vi "9213_UI.vi"(8 "error in (no error)":errorcluster, 11 "Node Ptr":T5 format="%.0x") -> (0 "error out":errorcluster)   [LabVIEW 2019, in "Modules.lvlib" / "9213.lvclass"]
uses:
  9213.lvclass
  <vilib>/NI VeriStand/Custom Device API/Custom Device Item Ref.ctl
  RSI Module/SubPanel Command.ctl
  Channels Listbox.ctl
  Thermocouple Type.ctl
  Measurement Units.ctl
  Conversion Time.ctl
  C:/Users/nitest/Desktop/Git 2019/niveristand-scan-engine-module-libraries/Source/RSI Module/RSI Module.lvclass
  9213.lvclass/9213.ctl
  RSI Module/RSI Module.lvclass
  <vilib>/NI VeriStand/Custom Device API/Custom Device API.lvlib
panel:
  in  "OTDComp":bool
  in  "Conversion Time":T1=1 items=["High Speed", "High Resolution"]
  in  "Units":T2 caption="Measurement Units" items=["Raw Volts", "Degrees Kelvin", "Degrees Celsius", "Degrees Fahrenheit", "Degrees Rankine"]
  in  "Type":T3 caption="Thermocouple Type" items=["J", "K", "T", "E", "R", "S", "N", "B"]
  in  "Channels":T4=[0]
  in  "SubPanel Event":refnum<user-event>
  in  "Header":cluster{"Section Name":string}={"Section Name"="NI 9205 Settings"}
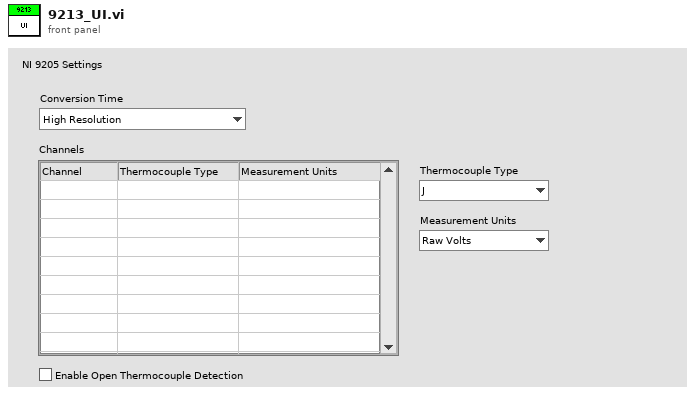
[diagram p1: front panel]
types:
  T1 = typedef "Modules.lvlib/9213.lvclass/Conversion Time.ctl" = u16
  T2 = typedef "Modules.lvlib/9213.lvclass/Measurement Units.ctl" = u8
  T3 = typedef "Modules.lvlib/9213.lvclass/Thermocouple Type.ctl" = u8
  T4 = typedef "Modules.lvlib/9213.lvclass/Channels Listbox.ctl" = i32[]
  T5 = typedef "Custom Device API.lvlib/Custom Device Item Ref.ctl" = u64
  T6 = typedef "Modules.lvlib/RSI Module.lvclass/Module Models.ctl" = enum16{"Empty", "NI 9201", "NI 9203", "NI 9205", "NI 9206", "NI 9207", "NI 9208", "NI 9209", "NI 9210", "NI 9211", "NI 9212", "NI 9213", "NI 9214", "NI 9215", "NI 9216", "NI 9217", "NI 9219", "NI 9220", "NI 9221", "NI 9222", "NI 9223", "NI 9224", "NI 9225", "NI 9226", "NI 9227", "NI 9228", "NI 9229", "NI 9233", "NI 9234", "NI 9235", "NI 9236", "NI 9237", "NI 9239", "NI 9242", "NI 9244", "NI 9253", "NI 9263", "NI 9264", "NI 9265", "NI 9266", "NI 9269", "NI 9344", "NI 9350", "NI 9375", "NI 9401", "NI 9402", "NI 9403", "NI 9411", "NI 9421", "NI 9422", "NI 9423", "NI 9425", "NI 9426", "NI 9435", "NI 9436", "NI 9437", "NI 9472", "NI 9474", "NI 9475", "NI 9476", "NI 9477", "NI 9478", "NI 9481", "NI 9482", "NI 9485"}
  T7 = typedef "Modules.lvlib/RSI Module.lvclass/SubPanel Command.ctl" = enum16{"Stop"}
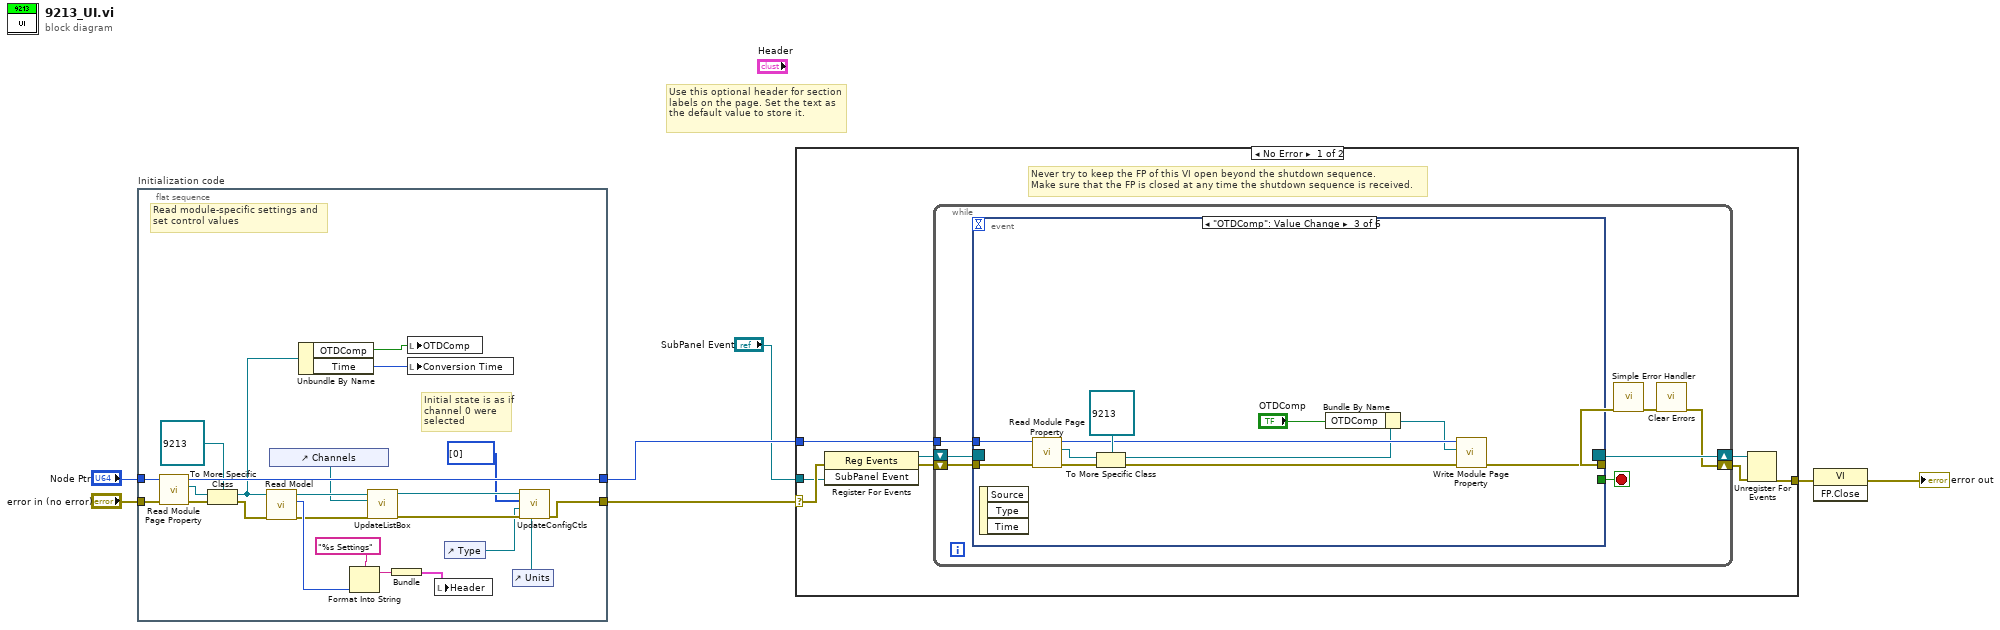
[diagram p0: block diagram]
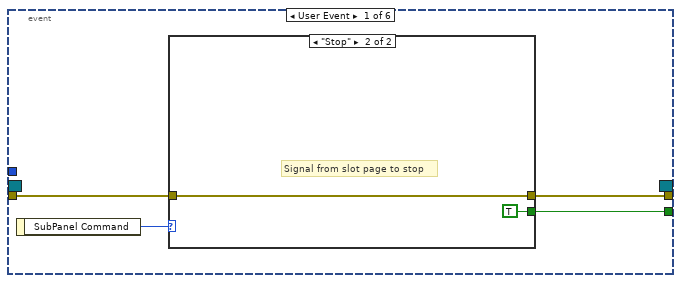
[diagram p2: hidden frame]
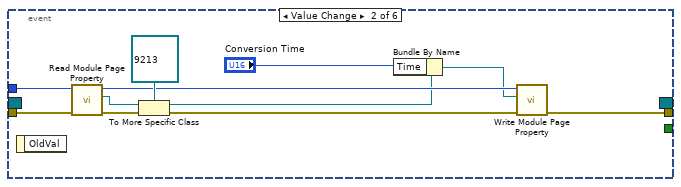
[diagram p4: hidden frame]
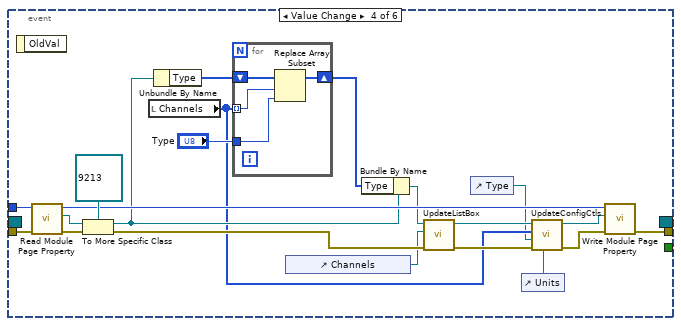
[diagram p5: hidden frame]
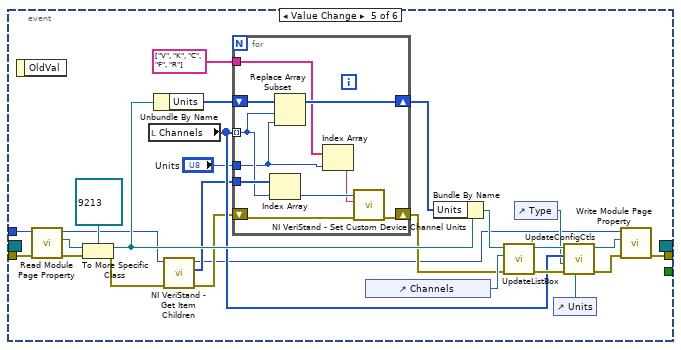
[diagram p6: hidden frame]
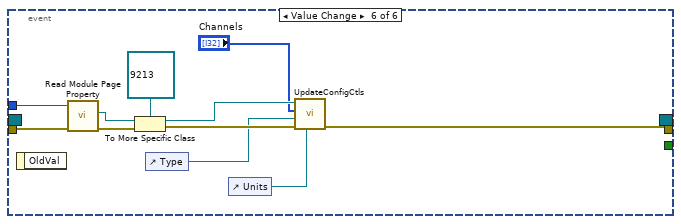
[diagram p7: hidden frame]
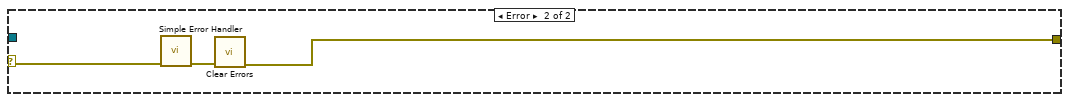
[diagram p8: hidden frame]
diagram:
  # "Use this optional header for section labels on the page. Set the text as the default value to store it."
  n1 = flat-sequence "Initialization code" {
    tunnel: "error in (no error)" -> [w29]
    tunnel: "Node Ptr" -> [w30]
    tunnel: [w12] -> w1
    tunnel: [w28] -> w4
    frame #0 {
      # "Initial state is as if channel 0 were selected"
      # "Read module-specific settings and\nset control values"
      n2 = call "Read Module Page Property.vi"("error in (no error)"=w29, "Node Ptr In"=w30) -> ("error out"=w27:errorcluster, "RSI Module"=w25:refnum<class "RSI Module.lvclass">, "Node Ptr Out"=w28:T5)  [unwired: 7 in]
      n3 = To More Specific Class(target class=refnum<class "9213.lvclass"> refnum ("9205 in"), reference=w25, error in=w27) -> (specific class reference=w15:refnum<class "9213.lvclass">, error out=w24:errorcluster)
      n4 = call "Read Model.vi"("error in (no error)"=w24, "RSI Module in"=w15) -> ("error out"=w18:errorcluster, "Model"=w22:T6, "RSI Module out"=w17:refnum<class "9213.lvclass">)  [unwired: 7 in]
      n5 = control-ref of="Channels"() -> (w16:refnum<vi>)
      n6 = Unbundle By Name(w15) -> ("OTDComp"=w8:bool, "Time"=w19:T1)
      n7 = Format Into String(format string="%s Settings", w22) -> (resulting string=w20:string)  [unwired: 2 in, 1 out]
      n8 = call "UpdateListBox.vi"("error in (no error)"=w18, "ListBox Refnum"=w16, "9213 in"=w17) -> ("error out"=w14:errorcluster, "9213 out"=w13:refnum<class "9213.lvclass">)  [unwired: 7 in]
      n9 = Bundle(w20) -> (w23:cluster{string})  [unwired: 1 in]
      n10 = local write "OTDComp"(w8) -> ()
      n11 = local write "Conversion Time"(w19) -> ()
      n12 = local write "Header"(w23) -> ()
      n13 = control-ref of="Type"() -> (w10:refnum<vi>)
      n14 = control-ref of="Units"() -> (w11:refnum<vi>)
      n15 = call "UpdateConfigCtls.vi"("Units"=w11, "error in (no error)"=w14, "Type"=w10, "Selected Channels"=T4 [0], "9213 in"=w13) -> ("error out"=w12:errorcluster)  [unwired: 5 in, 1 out]
    }
  }
  n16 = case shown="No Error" w1 {
    selector: w1 -> [w32 w150]
    tunnel: [w36 w148] -> w7
    tunnel: w4 -> [w33 _]
    tunnel: "SubPanel Event" -> [w31 _]
    frame No Error {
      # "Never try to keep the FP of this VI open beyond the shutdown sequence.\nMake sure that the FP is closed at any time the shutdown sequence is received."
      n17 = register-events(error in=w32, w31) -> (reference out=w34:refnum<event-registration>, error out=w35:errorcluster)  [unwired: 1 in]
      n18 = while {
        tunnel: w33 -> [w42]
        shift-right: [w39] -> w37
        shift-left: w35 -> [w45]
        shift-right: [w46] -> w38
        shift-left: w34 -> [w44]
        stop <- w43 stop-if-true
        n19 = event shown="[2] \"OTDComp\": Value Change" {
          selector: w44 -> [_ _ _ _ _ _]
          dyn-events: [_ _ _ _ _ _] -> w46
          timeout: _ -> [_ _ _ _ _ _]
          tunnel: w45 -> [w49 w58 w69 w91 w122 w144]
          tunnel: [w48 _ _ _ _ _] -> w43
          tunnel: [w47 w57 w68 w90 w121 w140] -> w41
          tunnel: w42 -> [_ w59 w70 w92 w123 w143]
          event User Event {
            n20 = event-data() -> ("SubPanel Command"=w50:T7)  [unwired: 1 out]
            n21 = case shown="\"Stop\"" w50 {
              tunnel: w49 -> [w51 w52]
              tunnel: [w51 w52] -> w47
              tunnel: [_ TRUE] -> w48
              frame Default {
              }
              frame "Stop" {
                # "Signal from slot page to stop"
              }
            }
          }
          event Value Change {
            n22 = event-data() -> ()  [unwired: 2 out]
            n23 = call "Read Module Page Property.vi"("error in (no error)"=w58, "Node Ptr In"=w59) -> ("error out"=w62:errorcluster, "RSI Module"=w63:refnum<class "RSI Module.lvclass">, "Node Ptr Out"=w60:T5)  [unwired: 7 in]
            n24 = To More Specific Class(target class=refnum<class "9213.lvclass"> refnum ("9205 in"), reference=w63, error in=w62) -> (specific class reference=w56:refnum<class "9213.lvclass">, error out=w61:errorcluster)
            n25 = Bundle By Name(cluster=w56, "Time"="Conversion Time") -> (w55:refnum<class "9213.lvclass">)
            n26 = call "Write Module Page Property.vi"("error in (no error)"=w61, "RSI Module"=w55, "Node Ptr In"=w60) -> ("error out"=w57:errorcluster)  [unwired: 6 in, 2 out]
          }
          event "OTDComp": Value Change {
            n27 = event-data() -> ()  [unwired: 4 out]
            n28 = call "Read Module Page Property.vi"("error in (no error)"=w69, "Node Ptr In"=w70) -> ("error out"=w73:errorcluster, "RSI Module"=w74:refnum<class "RSI Module.lvclass">, "Node Ptr Out"=w71:T5)  [unwired: 7 in]
            n29 = To More Specific Class(target class=refnum<class "9213.lvclass"> refnum ("9205 in"), reference=w74, error in=w73) -> (specific class reference=w67:refnum<class "9213.lvclass">, error out=w72:errorcluster)
            n30 = Bundle By Name(cluster=w67, "OTDComp"="OTDComp") -> (w66:refnum<class "9213.lvclass">)
            n31 = call "Write Module Page Property.vi"("error in (no error)"=w72, "RSI Module"=w66, "Node Ptr In"=w71) -> ("error out"=w68:errorcluster)  [unwired: 6 in, 2 out]
          }
          event Value Change {
            n32 = event-data() -> ()  [unwired: 2 out]
            n33 = call "Read Module Page Property.vi"("error in (no error)"=w91, "Node Ptr In"=w92) -> ("error out"=w94:errorcluster, "RSI Module"=w95:refnum<class "RSI Module.lvclass">, "Node Ptr Out"=w93:T5)  [unwired: 7 in]
            n34 = To More Specific Class(target class=refnum<class "9213.lvclass"> refnum ("9205 in"), reference=w95, error in=w94) -> (specific class reference=w85:refnum<class "9213.lvclass">, error out=w86:errorcluster)
            n35 = local read "Channels"() -> (w81:T4)
            n36 = Unbundle By Name(w85) -> ("Type"=w89:T3[])
            n37 = for {
              tunnel: w81 -> [w98] mode=indexing
              shift-right: [w99] -> w88
              shift-left: w89 -> [w100]
              tunnel: "Type" -> [w97]
              n38 = Replace Array Subset(array=w100, new element=w97, index=w98) -> (w99:T3[])
            }
            n39 = control-ref of="Channels"() -> (w80:refnum<vi>)
            n40 = Bundle By Name(cluster=w85, "Type"=w88) -> (w77:refnum<class "9213.lvclass">)
            n41 = call "UpdateListBox.vi"("error in (no error)"=w86, "ListBox Refnum"=w80, "9213 in"=w77) -> ("error out"=w84:errorcluster, "9213 out"=w82:refnum<class "9213.lvclass">)  [unwired: 7 in]
            n42 = control-ref of="Type"() -> (w78:refnum<vi>)
            n43 = control-ref of="Units"() -> (w79:refnum<vi>)
            n44 = call "UpdateConfigCtls.vi"("Units"=w79, "error in (no error)"=w84, "Type"=w78, "Selected Channels"=w81, "9213 in"=w82) -> ("error out"=w83:errorcluster, "9213 out"=w76:refnum<class "9213.lvclass">)  [unwired: 5 in]
            n45 = call "Write Module Page Property.vi"("error in (no error)"=w83, "RSI Module"=w76, "Node Ptr In"=w93) -> ("error out"=w90:errorcluster)  [unwired: 6 in, 2 out]
          }
          event Value Change {
            n46 = event-data() -> ()  [unwired: 2 out]
            n47 = call "Read Module Page Property.vi"("error in (no error)"=w122, "Node Ptr In"=w123) -> ("error out"=w124:errorcluster, "RSI Module"=w125:refnum<class "RSI Module.lvclass">, "Node Ptr Out"=w106:T5)  [unwired: 7 in]
            n48 = To More Specific Class(target class=refnum<class "9213.lvclass"> refnum ("9205 in"), reference=w125, error in=w124) -> (specific class reference=w118:refnum<class "9213.lvclass">, error out=w107:errorcluster)
            n49 = local read "Channels"() -> (w114:T4)
            n50 = Unbundle By Name(w118) -> ("Units"=w120:T2[])
            n51 = call <vilib>:"NI VeriStand - Get Item Children.vi"("error in (no error)"=w107, "Item Ref in"=w106) -> ("error out"=w104:errorcluster, "Child Refs"=w105:T5[], "Item Ref out"=w101:T5)  [unwired: 6 in, 1 out]
            n52 = for {
              tunnel: w114 -> [w133] mode=indexing
              shift-right: [w135] -> w119
              shift-left: w120 -> [w136]
              tunnel: "Units" -> [w128]
              shift-right: [w130] -> w103
              shift-left: w104 -> [w131]
              tunnel: w105 -> [w134]
              tunnel: string[] ["V", "K", "C", "F", "R"] -> [w129]
              n53 = Index Array(array=w134, index=w133) -> (element=w132:T5)
              n54 = Replace Array Subset(array=w136, new element=w128, index=w133) -> (w135:T2[])
              n55 = Index Array(array=w129, index=w128) -> (element=w127:string)
              n56 = call <vilib>:"NI VeriStand - Set Custom Device Channel Units.vi"("error in (no error)"=w131, "Units"=w127, "Channel Ref in"=w132) -> ("error out"=w130:errorcluster)  [unwired: 7 in, 1 out]
            }
            n57 = control-ref of="Channels"() -> (w113:refnum<vi>)
            n58 = Bundle By Name(cluster=w118, "Units"=w119) -> (w109:refnum<class "9213.lvclass">)
            n59 = call "UpdateListBox.vi"("error in (no error)"=w103, "ListBox Refnum"=w113, "9213 in"=w109) -> ("error out"=w117:errorcluster, "9213 out"=w115:refnum<class "9213.lvclass">)  [unwired: 7 in]
            n60 = control-ref of="Type"() -> (w110:refnum<vi>)
            n61 = control-ref of="Units"() -> (w112:refnum<vi>)
            n62 = call "UpdateConfigCtls.vi"("Units"=w112, "error in (no error)"=w117, "Type"=w110, "Selected Channels"=w114, "9213 in"=w115) -> ("error out"=w116:errorcluster, "9213 out"=w108:refnum<class "9213.lvclass">)  [unwired: 5 in]
            n63 = call "Write Module Page Property.vi"("error in (no error)"=w116, "RSI Module"=w108, "Node Ptr In"=w101) -> ("error out"=w121:errorcluster)  [unwired: 6 in, 2 out]
          }
          event Value Change {
            n64 = event-data() -> ()  [unwired: 2 out]
            n65 = call "Read Module Page Property.vi"("error in (no error)"=w144, "Node Ptr In"=w143) -> ("error out"=w145:errorcluster, "RSI Module"=w146:refnum<class "RSI Module.lvclass">)  [unwired: 7 in, 1 out]
            n66 = To More Specific Class(target class=refnum<class "9213.lvclass"> refnum ("9205 in"), reference=w146, error in=w145) -> (specific class reference=w141:refnum<class "9213.lvclass">, error out=w142:errorcluster)
            n67 = control-ref of="Type"() -> (w138:refnum<vi>)
            n68 = control-ref of="Units"() -> (w139:refnum<vi>)
            n69 = call "UpdateConfigCtls.vi"("Units"=w139, "error in (no error)"=w142, "Type"=w138, "Selected Channels"="Channels", "9213 in"=w141) -> ("error out"=w140:errorcluster)  [unwired: 5 in, 1 out]
          }
        }
        n70 = call <vilib>:"Simple Error Handler.vi"("error in (no error)"=w41) -> ("error out"=w40:errorcluster)  [unwired: 1 in, 7 out]
        n71 = call <vilib>:"Clear Errors.vi"("error in (no error)"=w40) -> ("error out"=w39:errorcluster)  [unwired: 1 in, 5 out]
      }
      n72 = Unregister For Events(event registration refnum=w38, error in=w37) -> (error out=w36:errorcluster)
    }
    frame Error {
      n73 = call <vilib>:"Simple Error Handler.vi"("error in (no error)"=w150) -> ("error out"=w149:errorcluster)  [unwired: 1 in, 7 out]
      n74 = call <vilib>:"Clear Errors.vi"("error in (no error)"=w149) -> ("error out"=w148:errorcluster)  [unwired: 1 in, 5 out]
    }
  }
  n75 = invoke class="VI" method="FP.Close"(error in=w7) -> (error out=→"error out":errorcluster)  [unwired: 2 in, 2 out]
